vi "get_target.vi"(2 "error in (no error)":errorcluster, 3 "Remote Server Address":string="palantir", 4 "Name":string) -> (0 "error out":errorcluster, 1 "CommonTargetData":T2)   [LabVIEW 2011]
uses:
  TCPdata.ctl
  TargetData.ctl
  CommonTargetData.ctl
panel:
  in  "Data":T1
  in  "Cluster":T3
  in  "Listen Port":u16=5311
  in  "Remote Server Port":u16=5310
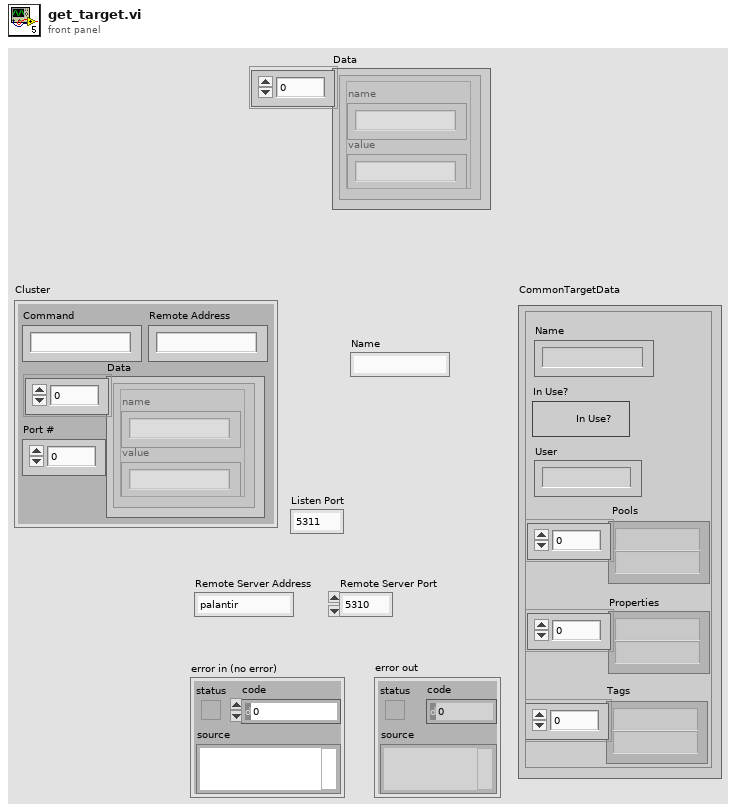
[diagram p1: front panel]
types:
  T1 = typedef "TargetData.ctl" = cluster{"name":string, "value":string}[]
  T2 = typedef "CommonTargetData.ctl" = cluster{"Name":string, "In Use?":bool, "User":string, " Pools":string[], "Tags":string[], "Properties":string[]}
  T3 = typedef "TCPdata.ctl" = cluster{"Data":T1, "Command":string, "Remote Address":string, "Port #":u16}
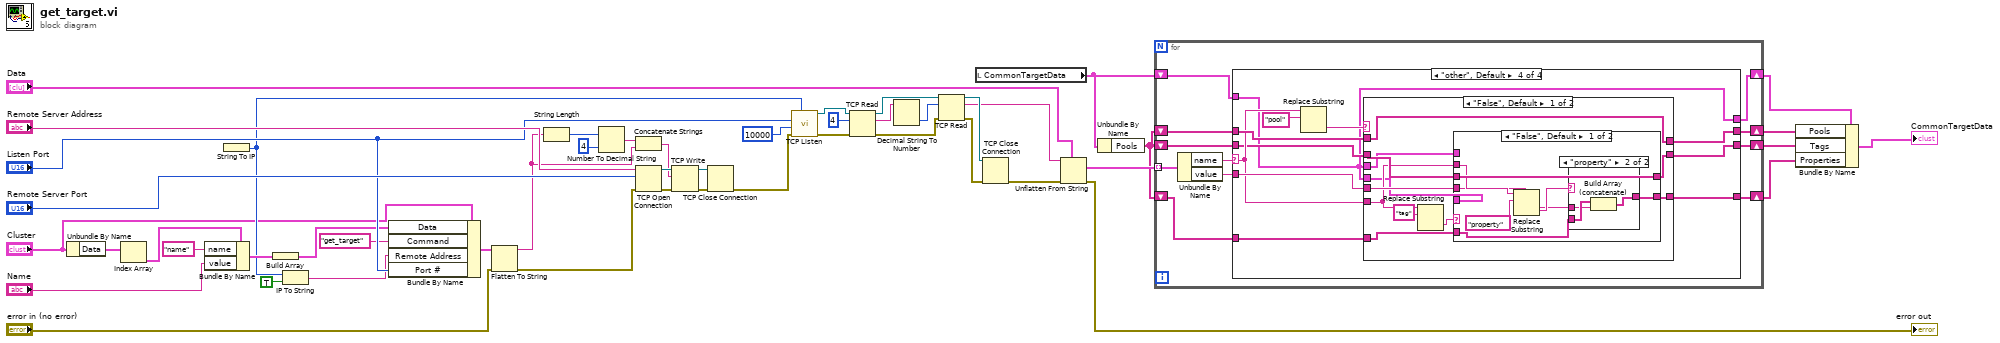
[diagram p0: block diagram]
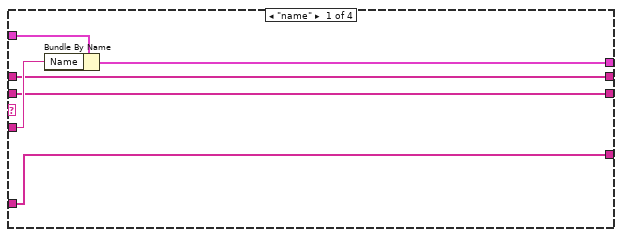
[diagram p2: hidden frame]
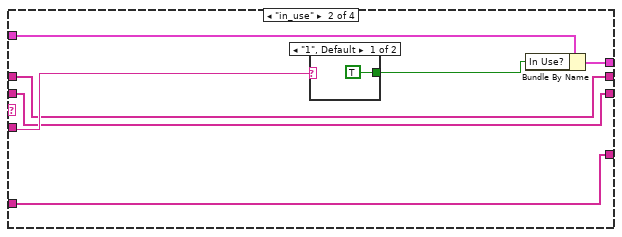
[diagram p3: hidden frame]
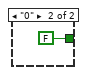
[diagram p4: hidden frame]
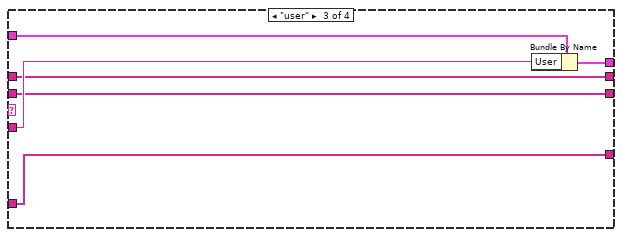
[diagram p5: hidden frame]
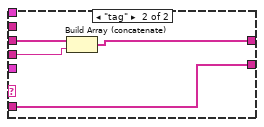
[diagram p7: hidden frame]
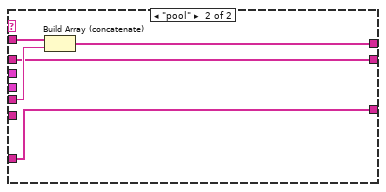
[diagram p8: hidden frame]
diagram:
  n1 = Unbundle By Name("Cluster") -> ("Data"=w35:T1)
  n2 = Index Array(array=w35) -> (element=w13:cluster{"name":string, "value":string})  [unwired: 1 in]
  n3 = Bundle By Name(cluster=w13, "name"="name", "value"="Name") -> (w34:cluster{"name":string, "value":string})
  n4 = String To IP() -> (0:w31:u32)  [unwired: 1 in]
  n5 = Build Array(w34) -> (w33:cluster{"name":string, "value":string}[])
  n6 = IP To String(1:TRUE ("dot notation? (F)"), 2:w31) -> (0:w37:string)
  n7 = Bundle By Name(cluster="Cluster", "Data"=w33, "Command"="get_target", "Remote Address"=w37, "Port #"="Listen Port") -> (w4:T3)
  n8 = Flatten To String(anything=w4, error in (no error)="error in (no error)") -> (data string=w26:string, error out=w24:errorcluster)  [unwired: 2 in, 1 out]
  n9 = String Length(string=w26) -> (length=w29:i32)
  n10 = Number To Decimal String(number=w29, width (-)=i16 4) -> (decimal integer string=w28:string)
  n11 = Concatenate Strings(w28, w26) -> (w30:string)
  n12 = TCP Open Connection(address="Remote Server Address", remote port or service name="Remote Server Port", error in (no error)=w24) -> (connection ID=w49:refnum<k5>, error out=w48:errorcluster)  [unwired: 2 out]
  n13 = TCP Write(connection ID=w49, data in=w30, error in (no error)=w48) -> (connection ID out=w46:refnum<k5>, error out=w47:errorcluster)  [unwired: 2 out]
  n14 = TCP Close Connection(connection ID=w46, error in (no error)=w47) -> (error out=w40:errorcluster)  [unwired: 2 out]
  n15 = call <vilib>:"TCP Listen.vi"("net address"=w31, "error in (no error)"=w40, "timeout ms (wait forever: -1)"=10000, "port"="Listen Port") -> ("error out"=w21:errorcluster, "connection ID"=w19:refnum<k5>)  [unwired: 3 in, 3 out]
  n16 = TCP Read(connection ID=w19, bytes to read=4, error in (no error)=w21) -> (connection ID out=w18:refnum<k5>, data out=w22:string, error out=w20:errorcluster)  [unwired: 1 in, 1 out]
  n17 = Decimal String To Number(string=w22) -> (number=w17:i32)  [unwired: 2 in, 1 out]
  n18 = TCP Read(connection ID=w18, bytes to read=w17, error in (no error)=w20) -> (connection ID out=w43:refnum<k5>, data out=w15:string, error out=w41:errorcluster)  [unwired: 1 in, 1 out]
  n19 = local read "CommonTargetData"() -> (w6:T2)
  n20 = TCP Close Connection(connection ID=w43, error in (no error)=w41) -> (error out=w16:errorcluster)  [unwired: 2 out]
  n21 = Unflatten From String(type="Data", binary string=w15, error in (no error)=w16) -> (value=w11:T1, error out=→"error out":errorcluster)  [unwired: 2 in, 1 out]
  n22 = Unbundle By Name(w6) -> ("Pools"=w2:string[])
  n23 = for {
    tunnel: w11 -> [w60] mode=indexing
    shift-right: [w56] -> w9
    shift-left: w6 -> [w57]
    shift-right: [w52] -> w5
    shift-left: w2 -> [w54]
    shift-right: [w53] -> w7
    shift-left: w2 -> [w55]
    shift-right: [w50] -> w1
    shift-left: w2 -> [w51]
    n24 = Unbundle By Name(w60) -> ("name"=w59:string, "value"=w58:string)
    n25 = case shown="\"other\", Default" w59 {
      selector: w59 -> [_ _ _ w88]
      tunnel: w58 -> [w64 w71 w79 w90]
      tunnel: w57 -> [w66 w73 w81 w84]
      tunnel: [w65 w72 w80 w84] -> w56
      tunnel: w55 -> [w63 w68 w77 w92]
      tunnel: w54 -> [w62 w69 w78 w86]
      tunnel: [w63 w68 w77 w91] -> w53
      tunnel: [w62 w69 w78 w85] -> w52
      tunnel: w51 -> [w61 w67 w76 w83]
      tunnel: [w61 w67 w76 w82] -> w50
      frame "name" {
        n26 = Bundle By Name(cluster=w66, "Name"=w64) -> (w65:T2)
      }
      frame "in_use" {
        n27 = case shown="\"1\", Default" w71 {
          tunnel: [TRUE ("In Use?") FALSE ("In Use?")] -> w70
          frame "1", Default {
          }
          frame "0" {
          }
        }
        n28 = Bundle By Name(cluster=w73, "In Use?"=w70) -> (w72:T2)
      }
      frame "user" {
        n29 = Bundle By Name(cluster=w81, "User"=w79) -> (w80:T2)
      }
      frame "other", Default {
        n30 = Replace Substring(4:"pool" ("substring (\"\")"), 5:w88) -> (0:w87:string)  [unwired: 2 in, 1 out]
        n31 = case shown="\"False\", Default" w87 {
          tunnel: w92 -> [w103 w123]
          tunnel: [w103 w122] -> w91
          tunnel: w90 -> [w100 w121]
          tunnel: w88 -> [w96 _]
          tunnel: w86 -> [w99 w120]
          tunnel: [w98 w120] -> w85
          tunnel: w84 -> [w97 _]
          tunnel: w84 -> [w95 _]
          tunnel: w83 -> [w94 w119]
          tunnel: [w93 w119] -> w82
          frame "False", Default {
            n32 = Replace Substring(4:"tag" ("substring (\"\")"), 5:w96) -> (0:w101:string)  [unwired: 2 in, 1 out]
            n33 = case shown="\"False\", Default" w101 {
              tunnel: w100 -> [w105 w117]
              tunnel: w99 -> [w110 w118]
              tunnel: [w110 w116] -> w98
              tunnel: w97 -> [_ _]
              tunnel: w96 -> [w106 _]
              tunnel: w95 -> [_ _]
              tunnel: w94 -> [w107 w115]
              tunnel: [w104 w115] -> w93
              frame "False", Default {
                n34 = Replace Substring(4:"property" ("substring (\"\")"), 5:w106) -> (0:w108:string)  [unwired: 2 in, 1 out]
                n35 = case shown="\"property\"" w108 {
                  tunnel: w107 -> [w111 w114]
                  tunnel: w105 -> [_ w113]
                  tunnel: [w111 w112] -> w104
                  frame "False", Default {
                  }
                  frame "property" {
                    n36 = Build Array (concatenate)(w114, w113) -> (w112:string[])
                  }
                }
              }
              frame "tag" {
                n37 = Build Array (concatenate)(w118, w117) -> (w116:string[])
              }
            }
          }
          frame "pool" {
            n38 = Build Array (concatenate)(w123, w121) -> (w122:string[])
          }
        }
      }
    }
  }
  n39 = Bundle By Name(cluster=w9, "Pools"=w7, "Tags"=w5, "Properties"=w1) -> (→"CommonTargetData":T2)
